vi "RSZVB Read Source Power Correction Data.vi"(7 "Calibrated Wave":string, 8 "error in (no error)":errorcluster {"code" format="%.0x"}, 9 "Port Number (1)":i32=1, 10 "Channel (1)":i32=1, 11 "VISA session":refnum<visa-resource-name>) -> (0 "error out":errorcluster {"code" format="%.0x"}, 2 "Power Correction Values":dbl[](array[numeric]) format="%^.3e", 3 "dup VISA session":refnum<visa-resource-name>)   [LabVIEW 2011]
doc: "This VI reads source power correction data sets. \n\nNote(s):\n\n(1) A power correction data set contains n real values. Each value corresponds to the ratio of the actual power at the reference plane (value provided by the used source) to the uncalibrated power in dB. \n\n(2) The number of values is equal to the number of sweep points.\n \n\nRemote-control command(s):\nSOURce<Ch>:POWer<Pt>:CORRection:DATA? '<src_string>'"
uses:
  _utility/RSZVB Global Data.vi
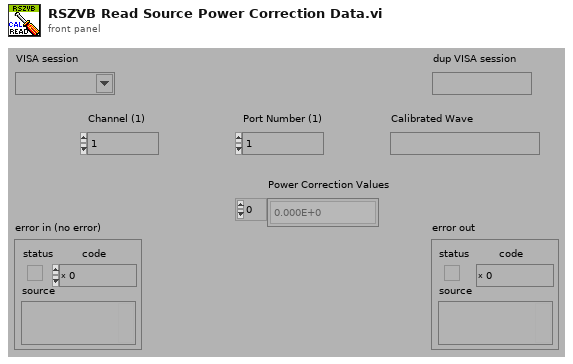
[diagram p1: front panel]
types:
  T1 = cluster{"Error Checking (T: On)":bool, "Installed Options":string[], "Data Valid?":bool, "Ports":i32, "Model":string[], "Option Checking (T: On)":bool}[]
  T2 = cluster{"Error Checking (T: On)":bool, "Installed Options":string[], "Data Valid?":bool, "Ports":i32, "Model":string[], "Option Checking (T: On)":bool}
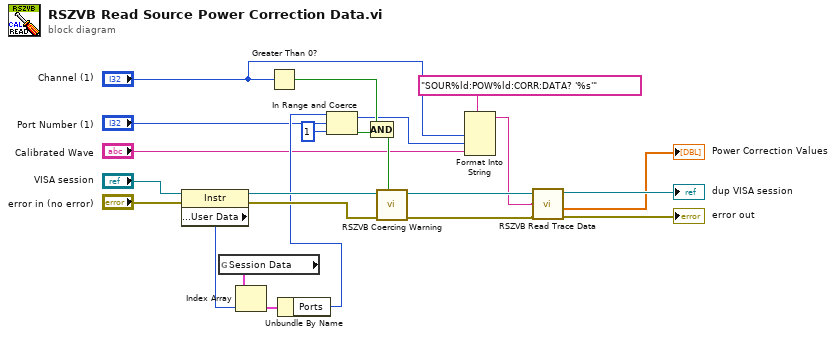
[diagram p0: block diagram]
diagram:
  n1 = property class="Instr"(reference="VISA session", error in="error in (no error)") -> (reference out=w17:refnum<visa-resource-name>, error out=w18:errorcluster, "General Settings:User Data"=w19:u32)
  n2 = global read "RSZVB Global Data.vi" "Session Data"() -> (w20:T1)
  n3 = Index Array(array=w20, index=w19) -> (element=w21:T2)
  n4 = Greater Than 0?(x="Channel (1)") -> (x > 0?=w23:bool)
  n5 = Unbundle By Name(w21) -> ("Ports"=w15:i32)
  n6 = In Range and Coerce(upper limit=w15, x="Port Number (1)", lower limit=1) -> (coerced(x)=w8:i32, In Range?=w14:bool)
  n7 = Compound Arithmetic op=AND(w23, w14) -> (w22:bool)
  n8 = call "RSZVB Coercing Warning.vi"("In Range?"=w22, "error in (no error)"=w18, "VISA session"=w17) -> ("error out"=w5:errorcluster, "dup VISA session"=w6:refnum<visa-resource-name>)  [unwired: 7 in]
  n9 = Format Into String(format string="SOUR%ld:POW%ld:CORR:DATA? '%s'", "Channel (1)", w8, "Calibrated Wave") -> (resulting string=w4:string)  [unwired: 2 in, 1 out]
  n10 = call "RSZVB Read Trace Data.vi"("error in (no error)"=w5, "Buffer"=w4, "VISA session"=w6) -> ("error out"=→"error out":errorcluster, "Trace Data"=→"Power Correction Values":dbl[], "dup VISA session"=→"dup VISA session":refnum<visa-resource-name>)  [unwired: 6 in]
